vi "NanotecSMCPD.constructor.vi"(0 "name":string, 2 "data in":string, 5 "error in (no error)":errorcluster) -> (14 "i ref out":refnum<vi>, 16 "data out":string, 19 "error out":errorcluster)   [LabVIEW 2014, in "NanotecSMCPD.lvlib"]
doc: "This is the constructor of a class.\n\nLicense Agreement for this software:\n\nCopyright (C)\nGesellschaft für Schwerionenforschung, GSI\nPlanckstr. 1\n64291 Darmstadt\nGermany\n\nContact: D.Beck@gsi.de \n\nThis program is free software; you can redistribute it and/or modify it under the terms of the \nGNU General Public License as published by the Free Software Foundation; either version 2 of \nthe license, or (at your option) any later version.\n\nThis program is distributed in the hope that it will be useful, but WITHOUT ANY WARRANTY; \nwithout even the implied warranty of MERCHANTABILITY or FITNESS FOR A PARTICULAR PURPOSE. See the GNU General License for more details (http://www.gnu.org).\n\nGesellschaft für Schwerionenforschung, GSI\nPlanckstr. 1, 64291 Darmstadt, Germany\nFor all questions and ideas contact: M.Richter@gsi.de, H.Brand@gsi.de or D.Beck@gsi.de.\nLast update: 16-JUN-2004"
uses:
  NanotecSMCPD.lvlib
  CS_Core/CSApplicationBaseClasses/DeviceBase/DeviceBase.myEventNames.ctl
  CS_Core/CSApplicationBaseClasses/MotorBase/MotorBase.myEventNames.ctl
  CSlibraries/UtilityLib/UtilityLib.valueStatus.ctl
  CS_Core/CSSystem/CSSystemLib/CSSystemLib.lvlib
  CS_Core/CSApplicationBaseClasses/MotorBase/MotorBase.lvlib
  CS_Core/CSApplicationBaseClasses/DeviceBase/DeviceBase.lvlib
  CSlibraries/UtilityLib/UtilityLib.lvlib
  CSlibraries-extern/DimLVEvent/LVDimInterface/LVDimInterface.lvlib
  CS_Core/CSSystem/CoreLib/CoreLib.lvlib
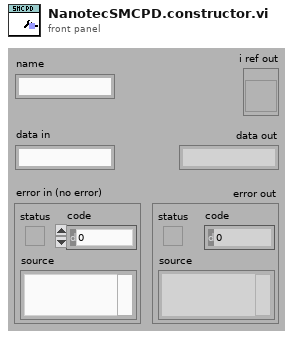
[diagram p1: front panel]
types:
  T1 = typedef "UtilityLib.lvlib/UtilityLib.valueStatus.ctl" = enum16{"no info available", "stand by/off", "on", "warning", "alarm/malfunction", "not implemented", "user action required", "important information", "system default", "control default", "indicator default", "button default"}
  T2 = enum16{"SetAttribute", "GetAttribute", "CreateAttribute", "DestroyAttribute", "DestroyAllAtributes"}
  T3 = cluster{"Method":enum16{"MoveRelative", "MoveAbsolute", "Stop"}, "Axis":i32, "Steps":dbl}
  T4 = typedef "MotorBase.lvlib/MotorBase.myEventNames.ctl" = enum16{"lvmsg://SetDefaultAxisIndex", "lvmsg://GetDefaultAxisIndex", "lvmsg://GetNofAxes", "lvmsg://EmergencyOff", "lvmsg://SetOnOff", "lvmsg://GetOnOff", "lvmsg://SetStartVelocity", "lvmsg://GetStartVelocity", "lvmsg://SetStopVelocity", "lvmsg://GetStopVelocity", "lvmsg://SetAcceleration", "lvmsg://GetAcceleration", "lvmsg://SetRangeMin", "lvmsg://GetRangeMin", "lvmsg://SetRangeMax", "lvmsg://GetRangeMax", "lvmsg://GetStatus", "lvmsg://SetPosition", "lvmsg://GetPosition", "lvmsg://GetNames", "lvmsg://GetUnit", "lvmsg://ResetDefault", "lvmsg://MoveAbsolute", "lvmsg://MoveRelative", "lvmsg://Stop", "lvmsg://Halt", "lvmsg://FindReference", "lvmsg://SetAxisOnOff", "lvmsg://GetAxisOnOff", "lvmsg://SetAxisStartVelocity", "lvmsg://GetAxisStartVelocity", "lvmsg://SetAxisStopVelocity", "lvmsg://GetAxisStopVelocity", "lvmsg://SetAxisAcceleration", "lvmsg://GetAxisAcceleration", "lvmsg://SetAxisRangeMin", "lvmsg://GetAxisRangeMin", "lvmsg://SetAxisRangeMax", "lvmsg://GetAxisRangeMax", "lvmsg://GetAxisStatus", "lvmsg://SetAxisPosition", "lvmsg://GetAxisPosition", "lvmsg://GetAxisNames", "lvmsg://GetAxisUnit", "lvmsg://ResetAxis", "lvmsg://MoveAxisAbsolute", "lvmsg://MoveAxisRelative", "lvmsg://StopAxis", "lvmsg://HaltAxis", "lvmsg://FindAxisReference"}
  T5 = typedef "DeviceBase.lvlib/DeviceBase.myEventNames.ctl" = enum16{"lvmsg://Initialize", "lvmsg://Close", "lvmsg://Configure", "lvmsg://Reset", "lvmsg://IDQuery"}
  T6 = typedef "NanotecSMCPD.lvlib/NanotecSMCPD.i attribute.ctl" = cluster{"referencing":bool[], "stop":bool[], "AutoHalt ID":i32, "MethodQueue":refnum<queue>, "Referenced1Time?":bool[], "LastCommand ID":i32}
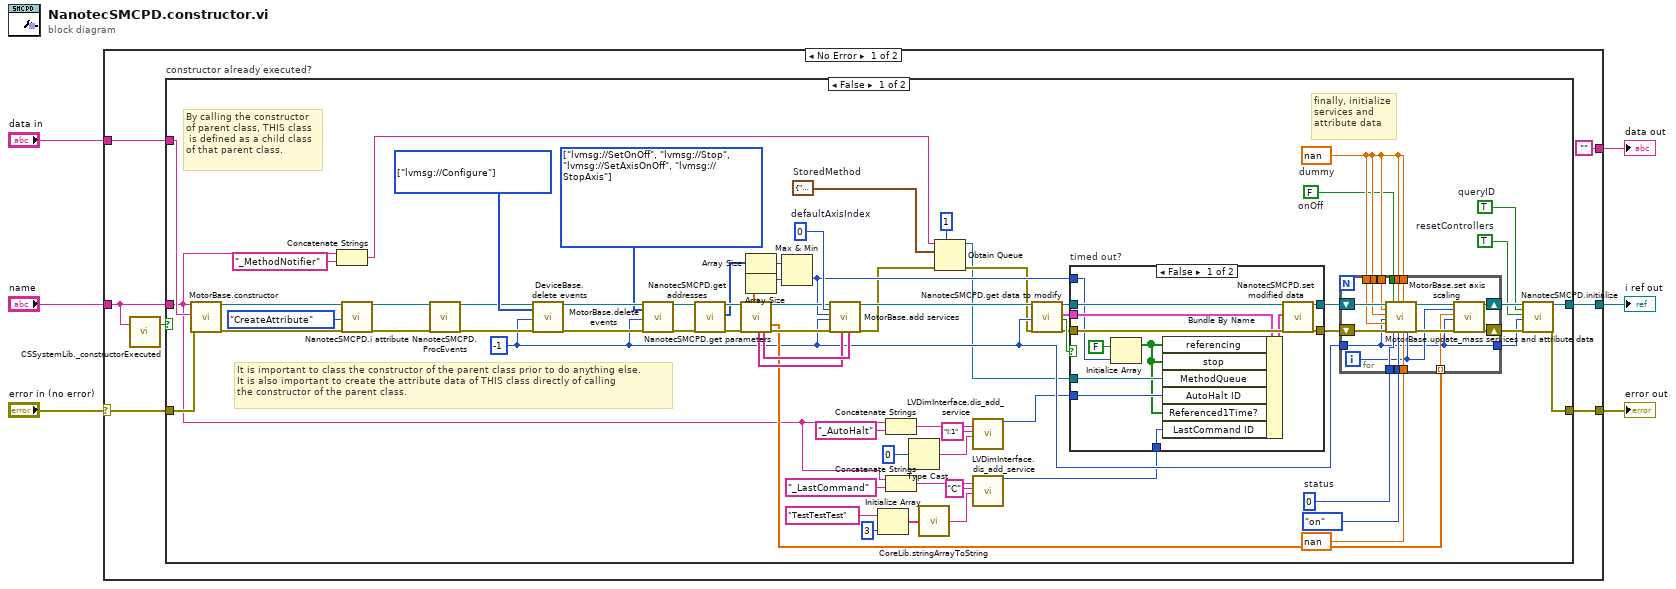
[diagram p0: block diagram]
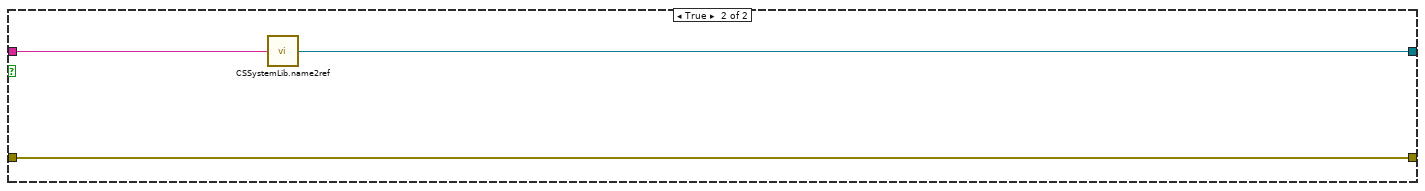
[diagram p3: hidden frame]
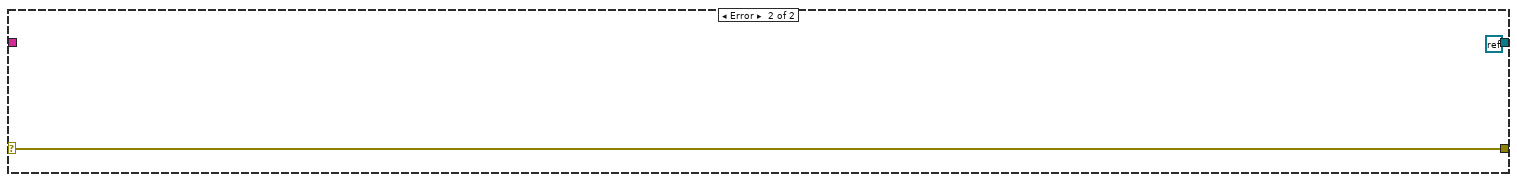
[diagram p4: hidden frame]
diagram:
  n1 = case shown="No Error" "error in (no error)" {
    selector: "error in (no error)" -> [w11 w119]
    tunnel: "name" -> [w10 _]
    tunnel: [w13 refnum<k0> refnum] -> w5
    tunnel: [w12 w119] -> w4
    tunnel: "data in" -> [w8 _]
    tunnel: ["" _] -> w1
    frame No Error {
      n2 = call "CSSystemLib._constructorExecuted.vi"("name"=w10) -> ("constructor executed?"=w9:bool)  [unwired: 18 in]
      n3 = case "constructor already executed?" shown="False" w9 {
        tunnel: w10 -> [w19 w118]
        tunnel: [w49 w117] -> w13
        tunnel: [w50 w116] -> w12
        tunnel: w11 -> [w78 w116]
        tunnel: w8 -> [w77 _]
        frame False {
          w35 = T3 {"Method"=enum."MoveRelative", "Axis"=0, "Steps"=0.0}  # StoredMethod
          w58 = nan  # dummy
          w71 = T4[] [enum."lvmsg://SetOnOff", enum."lvmsg://Stop", enum."lvmsg://SetAxisOnOff", enum."lvmsg://StopAxis"] items=["lvmsg://SetDefaultAxisIndex", "lvmsg://GetDefaultAxisIndex", "lvmsg://GetNofAxes", "lvmsg://EmergencyOff", "lvmsg://SetOnOff", "lvmsg://GetOnOff", "lvmsg://SetStartVelocity", "lvmsg://GetStartVelocity", "lvmsg://SetStopVelocity", "lvmsg://GetStopVelocity", "lvmsg://SetAcceleration", "lvmsg://GetAcceleration", "lvmsg://SetRangeMin", "lvmsg://GetRangeMin", "lvmsg://SetRangeMax", "lvmsg://GetRangeMax", "lvmsg://GetStatus", "lvmsg://SetPosition", "lvmsg://GetPosition", "lvmsg://GetNames", "lvmsg://GetUnit", "lvmsg://ResetDefault", "lvmsg://MoveAbsolute", "lvmsg://MoveRelative", "lvmsg://Stop", "lvmsg://Halt", "lvmsg://FindReference", "lvmsg://SetAxisOnOff", "lvmsg://GetAxisOnOff", "lvmsg://SetAxisStartVelocity", "lvmsg://GetAxisStartVelocity", "lvmsg://SetAxisStopVelocity", "lvmsg://GetAxisStopVelocity", "lvmsg://SetAxisAcceleration", "lvmsg://GetAxisAcceleration", "lvmsg://SetAxisRangeMin", "lvmsg://GetAxisRangeMin", "lvmsg://SetAxisRangeMax", "lvmsg://GetAxisRangeMax", "lvmsg://GetAxisStatus", "lvmsg://SetAxisPosition", "lvmsg://GetAxisPosition", "lvmsg://GetAxisNames", "lvmsg://GetAxisUnit", "lvmsg://ResetAxis", "lvmsg://MoveAxisAbsolute", "lvmsg://MoveAxisRelative", "lvmsg://StopAxis", "lvmsg://HaltAxis", "lvmsg://FindAxisReference"] ("events")
          w76 = T5[] [enum."lvmsg://Configure"] items=["lvmsg://Initialize", "lvmsg://Close", "lvmsg://Configure", "lvmsg://Reset", "lvmsg://IDQuery"] ("events")
          w47 = TRUE  # resetControllers
          w48 = TRUE  # queryID
          w57 = 0  # status
          w54 = FALSE  # onOff
          w62 = 0  # defaultAxisIndex
          w36 = -1 ("ms timeout (10000)")
          # "finally, initialize\nservices and\nattribute data"
          # "It is important to class the constructor of the parent class prior to do anything else.\nIt is also important to create the attribute data of THIS class directly of calling\nthe constructor of the parent class."
          # "By calling the constructor\nof parent class, THIS class\n is defined as a child class\nof that parent class."
          n4 = call "MotorBase.constructor.vi"("name"=w19, "data in"=w77, "error in (no error)"=w78) -> ("i ref out"=w83:refnum<vi>, "error out"=w82:errorcluster)  [unwired: 14 in, 1 out]
          n5 = Concatenate Strings(w19, "_MethodNotifier" ("string")) -> (w32:string)
          n6 = call "NanotecSMCPD.i attribute.vi"("VI Refnum"=w83, "Action"=T2."CreateAttribute", "error in (no error)"=w82) -> ("VI Refnum out"=w80:refnum<vi>, "error out"=w79:errorcluster)  [unwired: 14 in, 1 out]
          n7 = call "NanotecSMCPD.ProcEvents.vi"("i ref in"=w80, "error in (no error)"=w79) -> ("i ref out"=w75:refnum<vi>, "error out"=w74:errorcluster)  [unwired: 16 in]
          n8 = call "DeviceBase.delete events.vi"("i ref in"=w75, "events"=w76, "ms timeout (10000)"=w36, "error in (no error)"=w74) -> ("i ref out"=w72:refnum<vi>, "error out"=w73:errorcluster)  [unwired: 13 in, 1 out]
          n9 = call "MotorBase.delete events.vi"("i ref in"=w72, "events"=w71, "ms timeout (10000)"=w36, "error in (no error)"=w73) -> ("i ref out"=w70:refnum<vi>, "error out"=w69:errorcluster)  [unwired: 13 in, 1 out]
          n10 = call "NanotecSMCPD.get addresses.vi"("i ref in"=w70, "error in (no error)"=w69) -> ("i ref out"=w68:refnum<vi>, "controllerAddresses"=w63:i32[], "error out"=w67:errorcluster)  [unwired: 15 in]
          n11 = call "NanotecSMCPD.get parameters.vi"("i ref in"=w68, "error in (no error)"=w67) -> ("startFrequency [unit/s]"=w64:dbl[], "name"=w59:string[], "unit"=w60:string[], "i ref out"=w45:refnum<vi>, "scaling [unit]"=w53:dbl[], "error out"=w61:errorcluster)  [unwired: 6 in, 6 out]
          n12 = Array Size(array=w63) -> (size(s)=w65:i32)
          n13 = Array Size(array=w64) -> (size(s)=w66:i32)
          n14 = Max & Min(x=w65, y=w66) -> (min(x,y)=w37:i32)  [unwired: 1 out]
          n15 = call "MotorBase.add services.vi"("i ref in"=w45, "defaultAxisIndex"=w62, "nofAxes"=w37, "ms timeout (10000)"=w36, "error in (no error)"=w61, "logicalNames"=w59, "units"=w60) -> ("i ref out"=w44:refnum<vi>, "error out"=w34:errorcluster)  [unwired: 10 in, 1 out]
          n16 = Initialize Array("TestTestTest", 3 ("dimension size")) -> (w15:string[])
          n17 = Concatenate Strings(w19, "_AutoHalt" ("string")) -> (w27:string)
          n18 = Concatenate Strings(w19, "_LastCommand" ("string")) -> (w22:string)
          n19 = Type Cast(x=0) -> (*(type *) &x=w28:string)  [unwired: 1 in]
          n20 = call "CoreLib.stringArrayToString.vi"("Array"=w15) -> ("String"=w14:string)
          n21 = Obtain Queue(max queue size (-1, unlimited)=1, name (unnamed)=w32, element data type=w35, error in (no error)=w34) -> (queue out=w30:refnum<queue>, error out=w33:errorcluster)  [unwired: 1 in, 1 out]
          n22 = call "LVDimInterface.dis_add_service.vi"("serviceName"=w27, "typeDescriptor"="I:1", "data"=w28) -> ("my_serviceID"=w24:i32)  [unwired: 15 in, 1 out]
          n23 = call "LVDimInterface.dis_add_service.vi"("serviceName"=w22, "typeDescriptor"="C", "data"=w14) -> ("my_serviceID"=w18:i32)  [unwired: 15 in, 1 out]
          n24 = call "NanotecSMCPD.get data to modify.vi"("i ref in"=w44, "ms timeout (10000)"=w36, "error in (no error)"=w33) -> ("i ref out"=w40:refnum<vi>, "i attribute"=w38:T6, "timed out"=w43:bool, "error out"=w42:errorcluster)  [unwired: 13 in]
          n25 = case "timed out?" shown="False" w43 {
            tunnel: [w93 w97] -> w41
            tunnel: w42 -> [w92 w97]
            tunnel: [w94 w96] -> w39
            tunnel: w40 -> [w95 w96]
            tunnel: w38 -> [w91 _]
            tunnel: w37 -> [w89 _]
            tunnel: w30 -> [w87 _]
            tunnel: w24 -> [w86 _]
            tunnel: w18 -> [w84 _]
            frame False {
              n26 = Initialize Array(FALSE, w89) -> (w85:bool[])
              n27 = Bundle By Name(cluster=w91, "referencing"=w85, "stop"=w85, "MethodQueue"=w87, "AutoHalt ID"=w86, "Referenced1Time?"=w85, "LastCommand ID"=w84) -> (w90:T6)
              n28 = call "NanotecSMCPD.set modified data.vi"("i ref in"=w95, "i attribute"=w90, "error in (no error)"=w92) -> ("i ref out"=w94:refnum<vi>, "error out"=w93:errorcluster)  [unwired: 15 in]
            }
            frame True {
            }
          }
          n29 = for {
            shift-right: [w102] -> w51
            shift-left: w41 -> [w115]
            tunnel: w36 -> [w98]
            tunnel: w54 -> [w113]
            tunnel: w58 -> [w112]
            tunnel: w58 -> [w111]
            tunnel: w58 -> [w110]
            tunnel: w58 -> [w109]
            tunnel: w58 -> [w108]
            tunnel: w57 -> [w107]
            tunnel: UtilityLib.valueStatus."on" ("valueStatus") -> [w106]
            tunnel: nan ("position") -> [w101]
            tunnel: w53 -> [w99] mode=indexing
            shift-right: [w104] -> w52
            shift-left: w39 -> [w114]
            tunnel: [w98] -> w46
            i -> [w100]
            n30 = call "MotorBase.update_mass services and attribute data.vi"("i ref in"=w114, "acceleration"=w110, "rangeMin"=w109, "ms timeout (10000)"=w98, "rangeMax"=w108, "error in (no error)"=w115, "onOff"=w113, "status"=w107, "startVelocity"=w112, "valueStatus"=w106, "stopVelocity"=w111, "position"=w101, "axisNumber"=w100) -> ("i ref out"=w105:refnum<vi>, "error out"=w103:errorcluster)  [unwired: 4 in, 1 out]
            n31 = call "MotorBase.set axis scaling.vi"("i ref in"=w105, "axis"=w100, "scaling"=w99, "ms timeout (10000)"=w98, "error in (no error)"=w103) -> ("i ref out"=w104:refnum<vi>, "error out"=w102:errorcluster)  [unwired: 12 in, 1 out]
          }
          n32 = call "NanotecSMCPD.initialize.vi"("i ref in"=w52, "queryID"=w48, "resetControllers"=w47, "ms timeout (10000)"=w46, "error in (no error)"=w51) -> ("i ref out"=w49:refnum<vi>, "error out"=w50:errorcluster)  [unwired: 11 in, 2 out]
        }
        frame True {
          n33 = call "CSSystemLib.name2ref.vi"("name"=w118) -> ("obj refnum"=w117:refnum<vi>)
        }
      }
    }
    frame Error {
    }
  }
  "i ref out" <- w5
  "error out" <- w4
  "data out" <- w1
